vi "4339 Create Ch.vi"(10 "Device port info":T1[](array[typedef]), 11 "taskNumberer":string) -> (0 "error out":errorcluster, 2 "Channels":string[](array[string]), 3 "taskCluster":T2)   [LabVIEW 2022 SP3]
uses:
  4339cluster.ctl
  <vilib>/DAQmx/create/channels.llb/DAQmx Create Channel (AI-Voltage-Basic).vi
  <vilib>/DAQmx/configure/timing.llb/DAQmx Timing (Sample Clock).vi
  <vilib>/DAQmx/create/channels.llb/DAQmx Create Channel (AI-Voltage-Custom with Excitation).vi
  Device ID port info.ctl
panel:
  out "FS 18":dbl
  out "Fs SG":dbl
  out "Slot 18 Task":refnum<k21>
  out "SG Tasks OUT":refnum<k21>[](array[refnum])
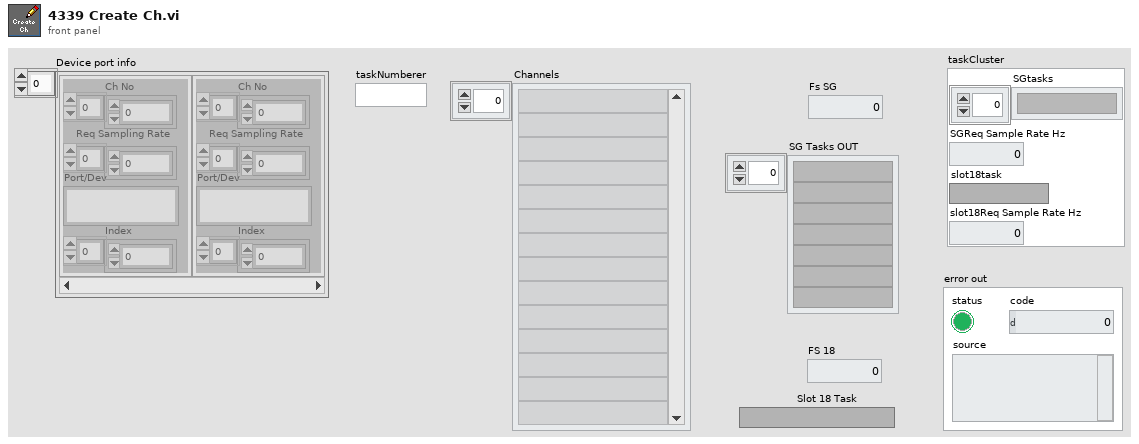
[diagram p1: front panel]
types:
  T1 = typedef "Device ID port info.ctl" = cluster{"Ch No":i16[], "Req Sampling Rate":dbl[], "Port":string, "Index":i32[]}
  T2 = typedef "4339cluster.ctl" = cluster{"SGtasks":refnum<k21>[], "SGReq Sample Rate Hz":dbl, "slot18task":refnum<k21>, "slot18Req Sample Rate Hz":dbl}
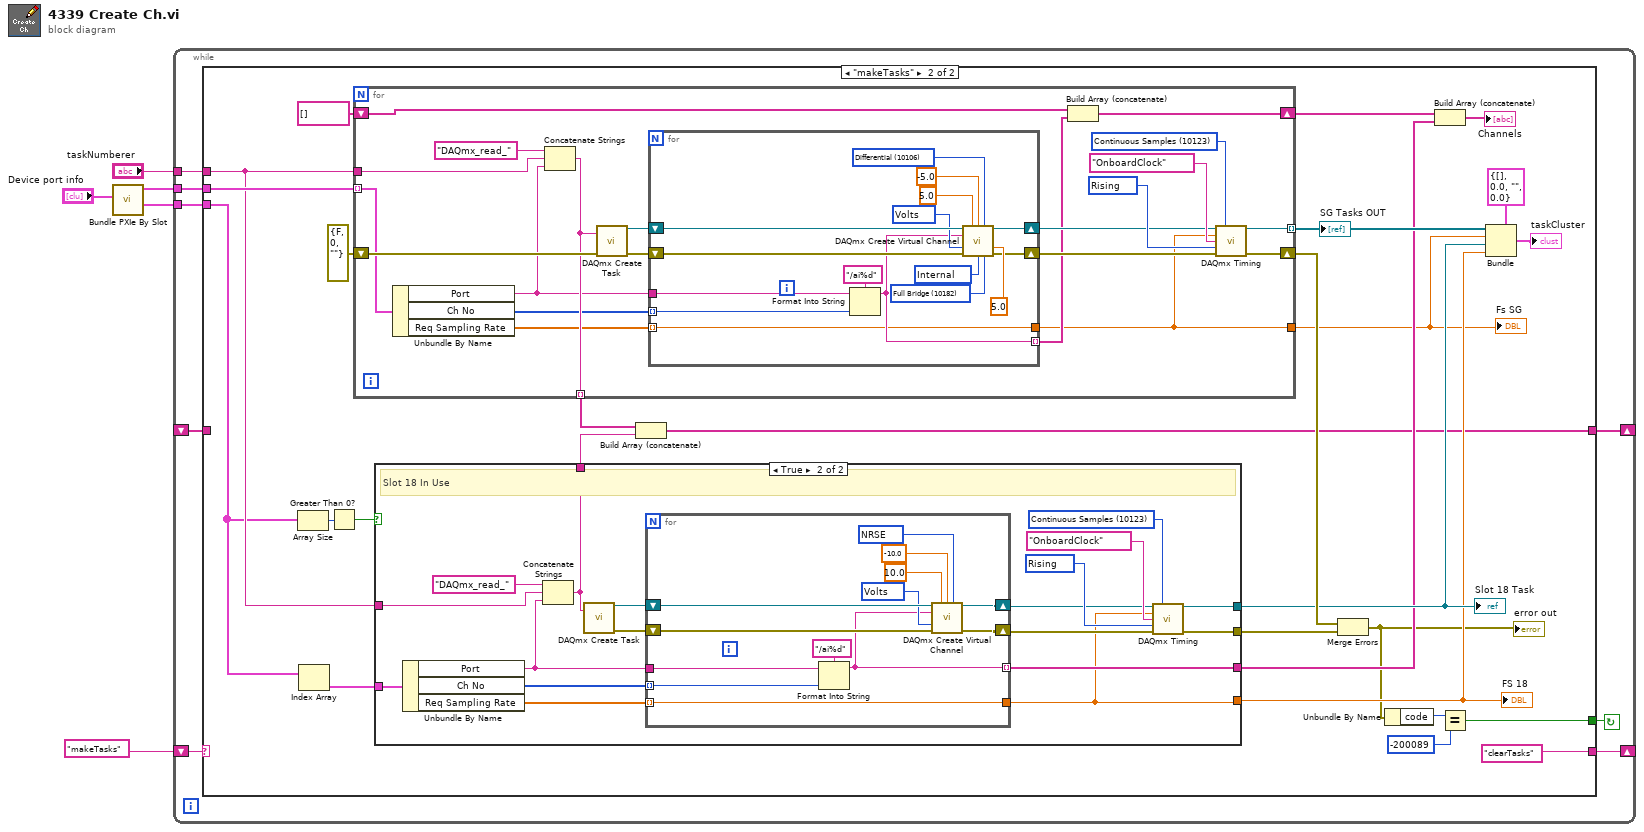
[diagram p0: block diagram]
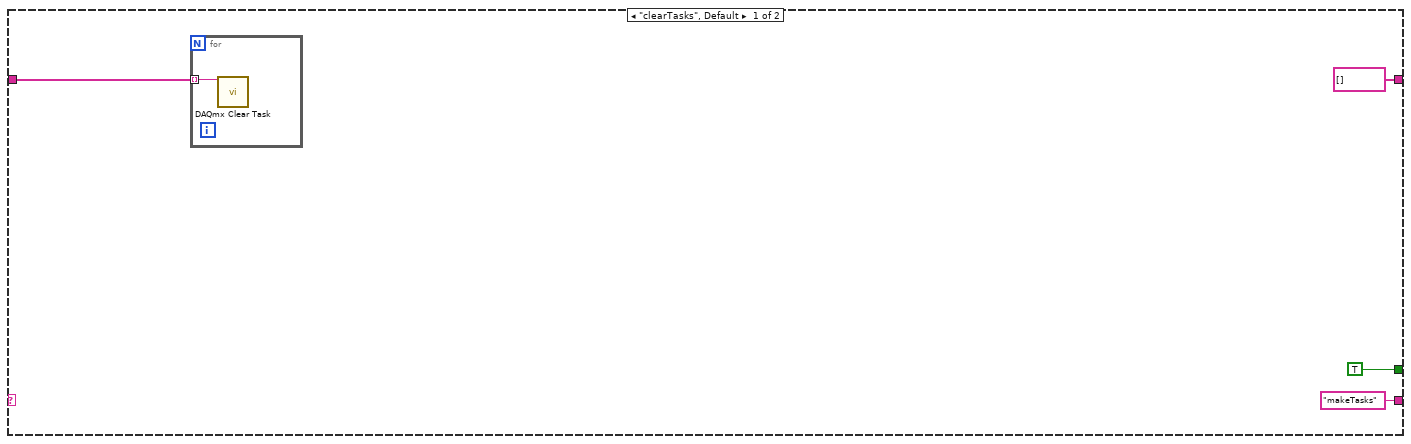
[diagram p2: hidden frame]
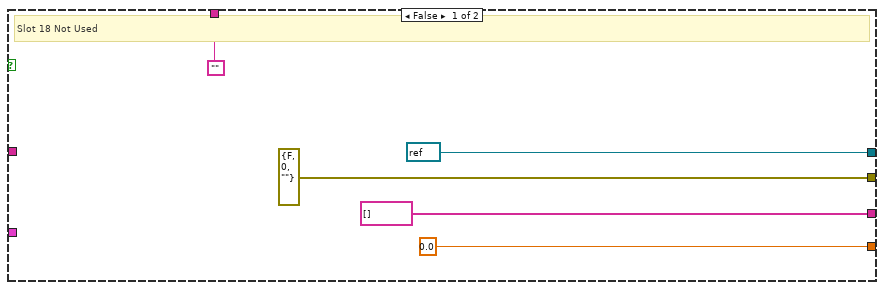
[diagram p3: hidden frame]
diagram:
  n1 = call "Bundle PXIe By Slot.vi"("Device port info"="Device port info") -> ("Slot18"=w1:T1[], "SGslots"=w5:T1[])  [unwired: 9 in]
  n2 = while {
    tunnel: w5 -> [w13]
    tunnel: "taskNumberer" -> [w12]
    tunnel: w1 -> [w11]
    shift-right: [w8] -> _
    shift-left: "makeTasks" -> [w9]
    shift-right: [w7] -> _
    shift-left: _ -> [w6]
    stop <- w10 continue-if-true
    n3 = case shown="\"makeTasks\"" w9 {
      tunnel: w13 -> [_ w45]
      tunnel: w12 -> [_ w43]
      tunnel: w11 -> [_ w42]
      tunnel: [TRUE w30] -> w10
      tunnel: ["makeTasks" "clearTasks"] -> w8
      tunnel: [string[] [] w22] -> w7
      tunnel: w6 -> [w16 _]
      frame "clearTasks", Default {
        n4 = for {
          tunnel: w16 -> [w18] mode=indexing
          n5 = call <vilib>:"DAQmx Clear Task.vi"("task in"=w18) -> ()  [unwired: 14 in, 1 out]
        }
      }
      frame "makeTasks" {
        n6 = Array Size(array=w42) -> (size(s)=w41:i32)
        n7 = Index Array(array=w42) -> (element=w19:T1)  [unwired: 1 in]
        n8 = Greater Than 0?(x=w41) -> (x > 0?=w40:bool)
        n9 = for {
          tunnel: w43 -> [w101]
          tunnel: w45 -> [w99] mode=indexing
          shift-right: [w91] -> w39
          shift-left: errorcluster {"status"=FALSE, "code"=0, "source"=""} ("error out") -> [w100]
          tunnel: [w90] -> w36 mode=indexing
          shift-right: [w88] -> w34
          shift-left: string[] [] -> [w87]
          tunnel: [w86] -> w26
          tunnel: [w85] -> w24 mode=indexing
          w94 = 10280 items=["Rising"=10280, "Falling"=10171] ("active edge")
          w96 = 10123 items=["Finite Samples"=10178, "Continuous Samples"=10123, "Hardware Timed Single Point"=12522] ("sample mode")
          n10 = Unbundle By Name(w99) -> ("Port"=w82:string, "Ch No"=w84:i16[], "Req Sampling Rate"=w83:dbl[])
          n11 = Concatenate Strings("DAQmx_read_" ("new task name"), w101, w82) -> (w85:string)
          n12 = call <vilib>:"DAQmx Create Task.vi"("new task name"=w85, "error in"=w100) -> ("task out"=w98:refnum<k21>, "error out"=w97:errorcluster)  [unwired: 3 in, 9 out]
          n13 = for {
            shift-right: [w107] -> w93
            shift-left: w98 -> [w117]
            shift-right: [w106] -> w92
            shift-left: w97 -> [w112]
            tunnel: [w108] -> w89 mode=indexing
            tunnel: [w103] -> w86
            tunnel: w82 -> [w105]
            tunnel: w84 -> [w104] mode=indexing
            tunnel: w83 -> [w103] mode=indexing
            w110 = 10182 items=["Full Bridge"=10182, "Half Bridge"=10187, "Quarter Bridge"=10270, "No Bridge"=10228] ("bridge configuration")
            w111 = 10200 items=["Internal"=10200, "External"=10167, "None"=10230] ("voltage excitation source")
            w113 = 10348 items=["Volts"=10348, "From Custom Scale"=10065] ("units")
            w116 = 10106 items=["Default"=-1, "RSE"=10083, "NRSE"=10078, "Differential"=10106, "Pseudodifferential"=12529] ("input terminal configuration")
            n14 = Format Into String(format string="/ai%d", initial string=w105, w104) -> (resulting string=w108:string)  [unwired: 1 in, 1 out]
            n15 = call-poly <vilib>:"DAQmx Create Virtual Channel.vi"("task in"=w117, "maximum value"=5.0, "minimum value"=-5.0, "input terminal configuration"=w116, "physical channels"=w108, "units"=w113, "voltage excitation value"=5.0, "error in"=w112, "voltage excitation source"=w111, "bridge configuration"=w110) -> ("task out"=w107:refnum<k21>, "error out"=w106:errorcluster)  [unwired: 3 in, 1 out]
          }
          n16 = Build Array (concatenate)(w87, w89) -> (w88:string[])
          n17 = call-poly <vilib>:"DAQmx Timing.vi"("task/channels in"=w93, "sample mode"=w96, "rate"=w86, "source"=tag "OnboardClock", "active edge"=w94, "error in"=w92) -> ("task out"=w90:refnum<k21>, "error out"=w91:errorcluster)  [unwired: 1 in, 7 out]
        }
        "SG Tasks OUT" <- w36
        "Fs SG" <- w26
        n18 = case shown="True" w40 {
          tunnel: w43 -> [_ w67]
          tunnel: [errorcluster {"status"=FALSE, "code"=0, "source"=""} ("error out") w60] -> w37
          tunnel: [refnum<k21> refnum ("task out") w59] -> w35
          tunnel: [0.0 ("Req Sample Rate Hz") w53] -> w27
          tunnel: [string[] [] w58] -> w33
          tunnel: ["" w56] -> w23
          tunnel: w19 -> [_ w52]
          frame False {
            # "Slot 18 Not Used"
          }
          frame True {
            w65 = 10280 items=["Rising"=10280, "Falling"=10171] ("active edge")
            w63 = 10123 items=["Finite Samples"=10178, "Continuous Samples"=10123, "Hardware Timed Single Point"=12522] ("sample mode")
            # "Slot 18 In Use"
            n19 = Unbundle By Name(w52) -> ("Port"=w51:string, "Ch No"=w55:i16[], "Req Sampling Rate"=w54:dbl[])
            n20 = Concatenate Strings("DAQmx_read_" ("new task name"), w67, w51) -> (w56:string)
            n21 = call <vilib>:"DAQmx Create Task.vi"("new task name"=w56) -> ("task out"=w66:refnum<k21>, "error out"=w57:errorcluster)  [unwired: 4 in, 9 out]
            n22 = for {
              shift-right: [w73] -> w62
              shift-left: w66 -> [w80]
              shift-right: [w72] -> w61
              shift-left: w57 -> [w75]
              tunnel: [w74] -> w58 mode=indexing
              tunnel: w51 -> [w71]
              tunnel: w55 -> [w70] mode=indexing
              tunnel: [w69] -> w53
              tunnel: w54 -> [w69] mode=indexing
              w76 = 10348 items=["Volts"=10348, "From Custom Scale"=10065] ("units")
              w79 = 10078 items=["Default"=-1, "RSE"=10083, "NRSE"=10078, "Differential"=10106, "Pseudodifferential"=12529] ("input terminal configuration")
              n23 = Format Into String(format string="/ai%d", initial string=w71, w70) -> (resulting string=w74:string)  [unwired: 1 in, 1 out]
              n24 = call-poly <vilib>:"DAQmx Create Virtual Channel.vi"("task in"=w80, "maximum value"=10.0, "minimum value"=-10.0, "input terminal configuration"=w79, "physical channels"=w74, "units"=w76, "error in"=w75) -> ("task out"=w73:refnum<k21>, "error out"=w72:errorcluster)  [unwired: 2 in, 5 out]
            }
            n25 = call-poly <vilib>:"DAQmx Timing.vi"("task/channels in"=w62, "sample mode"=w63, "rate"=w53, "source"=tag "OnboardClock", "active edge"=w65, "error in"=w61) -> ("task out"=w59:refnum<k21>, "error out"=w60:errorcluster)  [unwired: 1 in, 7 out]
          }
        }
        "Slot 18 Task" <- w35
        "FS 18" <- w27
        n26 = Build Array (concatenate)(w24, w23) -> (w22:string[])
        n27 = Merge Errors(w39, w37) -> (w25:errorcluster)
        "error out" <- w25
        n28 = Unbundle By Name(w25) -> ("code"=w32:i32)
        n29 = Build Array (concatenate)(w34, w33) -> (→"Channels":string[])
        n30 = Equal?(x=w32, y=-200089) -> (x = y?=w30:bool)
        n31 = Bundle(cluster=T2 {"SGtasks"=[], "SGReq Sample Rate Hz"=0.0, "slot18task"="", "slot18Req Sample Rate Hz"=0.0} ("taskCluster"), "SGtasks"=w36, "SGReq Sample Rate Hz"=w26, "slot18task"=w35, "slot18Req Sample Rate Hz"=w27) -> (→"taskCluster":T2)
      }
    }
  }
